vi "Run.vi"(8 "error in (no error)":errorcluster, 11 "SOL-Server in":refnum<class "SOL-Server.lvclass">) -> (0 "error out":errorcluster, 3 "SOL-Server out":refnum<class "SOL-Server.lvclass">)   [LabVIEW 2020, in "Summer of LabVIEW.lvlib" / "SOL-Server.lvclass"]
uses:
  SOL-Server.lvclass
  SOL-Server.lvclass/SOL-Server.ctl
  <vilib>/IlluminatedG/IG HTTP Server/HTTP Server/Server/Server.lvclass
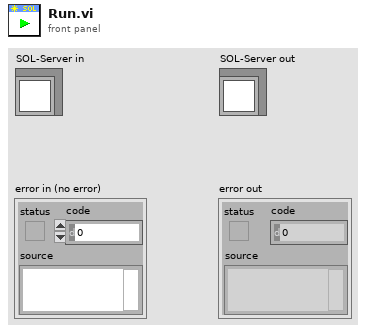
[diagram p1: front panel]
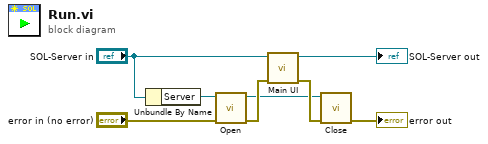
[diagram p0: block diagram]
diagram:
  n1 = Unbundle By Name("SOL-Server in") -> ("Server"=w7:refnum<class "Server.lvclass">)
  n2 = call <vilib>:"Open.vi"("error in (no error)"="error in (no error)", "Server in"=w7) -> ("error out"=w4:errorcluster, "Server out"=w3:refnum<class "Server.lvclass">)  [unwired: 8 in]
  n3 = call "Main UI.vi"("error in (no error)"=w4, "SOL-Server in"="SOL-Server in") -> ("error out"=w8:errorcluster, "SOL-Server out"=→"SOL-Server out":refnum<class "SOL-Server.lvclass">)  [unwired: 8 in]
  n4 = call <vilib>:"Close.vi"("error in (no error)"=w8, "Server in"=w3) -> ("error out"=→"error out":errorcluster)  [unwired: 8 in, 1 out]
